vi "Reset ROI.vi"(8 "error in":errorcluster, 11 "Base Graph in":refnum<class "Base Graph.lvclass">) -> (0 "error out":errorcluster, 3 "Base Graph out":refnum<class "Base Graph.lvclass">)   [LabVIEW 2023, in "Base Graph.lvclass"]
uses:
  Base Graph.lvclass
  Base Graph.lvclass/Base Graph.ctl
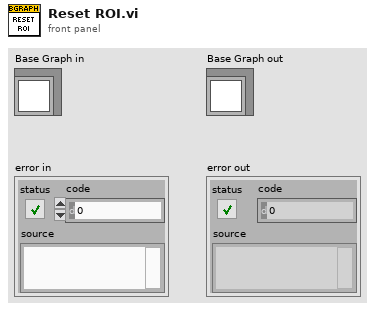
[diagram p1: front panel]
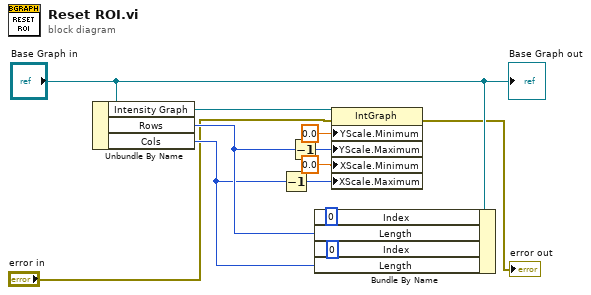
[diagram p0: block diagram]
diagram:
  n1 = Unbundle By Name("Base Graph in") -> ("Intensity Graph"=w11:refnum<vi>, "Rows"=w6:u32, "Cols"=w5:u32)
  n2 = Decrement(x=w5) -> (x-1=w3:u32)
  n3 = Decrement(x=w6) -> (x-1=w4:u32)
  n4 = Bundle By Name(cluster="Base Graph in", "Index"=u32 0 ("ROI XY.ROI X.Index"), "Length"=w6, "Index"=u32 0 ("ROI XY.ROI Y.Index"), "Length"=w5) -> ()  [unwired: 1 out]
  n5 = property class="IntGraph"(reference=w11, error in="error in", "YScale.Minimum"=0.0 ("Y Scale.Range:Minimum"), "YScale.Maximum"=w4, "XScale.Minimum"=0.0 ("X Scale.Range:Minimum"), "XScale.Maximum"=w3) -> (error out=→"error out":errorcluster)  [unwired: 1 out]
  "Base Graph out" <- "Base Graph in"
